vi "GetSgmtsOffsts.vi"(8 "error in":errorcluster, 11 "file path (use dialog)":path) -> (0 "error out":errorcluster, 1 "# of sgmts":i32, 2 "offsets":u64[](array[numeric]), 3 "path":path, 4 "Pass?":bool)   [LabVIEW 2016]
panel:
  out "Failed Lead In Data":u32[](array[numeric]) format="%.0x"
  out "TDMS segment":i32
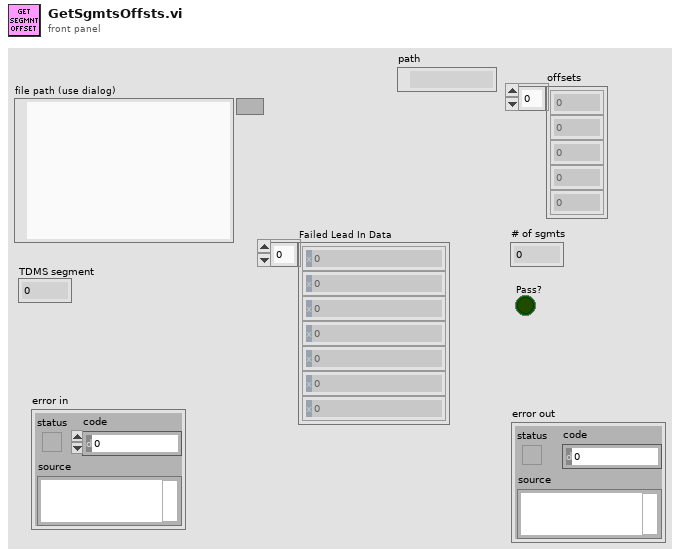
[diagram p1: front panel]
types:
  T1 = enum16{"big-endian, network order", "native, host order", "little-endian"}
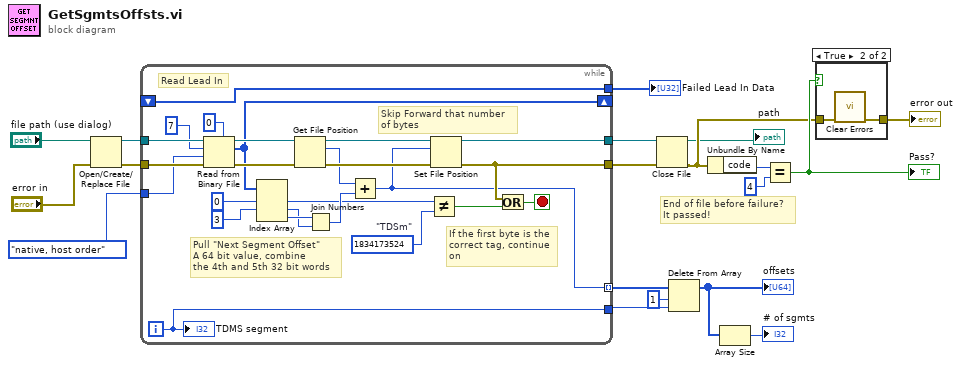
[diagram p0: block diagram]
diagram:
  # "End of file before failure?\nIt passed!"
  n1 = Open/Create/Replace File(file path (use dialog)="file path (use dialog)", error in="error in") -> (refnum out=w17:refnum<file>, error out=w18:errorcluster)  [unwired: 4 in, 1 out]
  n2 = while {
    tunnel: w18 -> [w44]
    tunnel: w17 -> [w43]
    tunnel: T1."native, host order" ("byte order (0:big-endian, network order)") -> [w42]
    tunnel: [w25] -> w15
    tunnel: [w32] -> w14
    shift-right: [w26] -> _
    shift-left: _ -> [w22]
    tunnel: [w22] -> w11
    tunnel: [w21] -> w10 mode=indexing
    tunnel: [w20] -> w8
    i -> [w20]
    stop <- w23 stop-if-true
    w27 = u32 1834173524  # "TDSm"
    # "If the first byte is the\ncorrect tag, continue\non"
    # "Read Lead In"
    # "Skip Forward that number\nof bytes"
    # "Pull \"Next Segment Offset\"\nA 64 bit value, combine\nthe 4th and 5th 32 bit words"
    n3 = Read from Binary File(5:u32 0, 8:w44, 9:w42, 10:7 ("count (1)"), 11:w43) -> (0:w35:errorcluster, 2:w26:u32[], 3:w36:refnum<file>)  [unwired: 1 in, 1 out]
    n4 = Index Array(array=w26, index #1=0 ("index"), index #2=3 ("index")) -> (element #1=w28:u32, element #2=w37:u32, element #3=w38:u32)  [unwired: 1 in]
    n5 = Get File Position(4:w35, 7:w36) -> (0:w34:errorcluster, 2:w31:i64, 3:w33:refnum<file>)
    n6 = Join Numbers(hi=w38, lo=w37) -> ((hi.lo)=w30:u64)
    n7 = Add(x=w31, y=w30) -> (x+y=w21:u64)
    n8 = Not Equal?(x=w28, y=w27) -> (x != y?=w24:bool)
    n9 = Set File Position(offset (in bytes) (0)=w21, refnum=w33, error in=w34) -> (refnum out=w32:refnum<file>, error out=w25:errorcluster)  [unwired: 1 in]
    n10 = Or(x=w25, y=w24) -> (x .or. y?=w23:bool)
    "TDMS segment" <- w20
  }
  "Failed Lead In Data" <- w11
  n11 = Close File(refnum=w14, error in=w15) -> (path=→"path":path, error out=w4:errorcluster)
  n12 = Delete From Array(array=w10, length=1, index=w8) -> (array with subset deleted=w7:u64[])  [unwired: 1 out]
  "offsets" <- w7
  n13 = Unbundle By Name(w4) -> ("code"=w13:i32)
  n14 = Array Size(array=w7) -> (size(s)=→"# of sgmts":i32)
  n15 = Equal?(x=w13, y=4) -> (x = y?=w5:bool)
  "Pass?" <- w5
  n16 = case shown="True" w5 {
    tunnel: w4 -> [w45 w47]
    tunnel: [w45 w46] -> w3
    frame False {
    }
    frame True {
      n17 = call <vilib>:"Clear Errors.vi"("error in (no error)"=w47) -> ("error out"=w46:errorcluster)  [unwired: 5 in, 1 out]
    }
  }
  "error out" <- w3
